vi "callTransport.vi"() -> ()   [LabVIEW 2019]
uses:
  <userlib>/LevyLab/Transport/Control Experiment/Control Experiment.lvclass/Control Experiment.ctl
  <userlib>/LevyLab/Transport/Transport/Transport.lvclass/Transport.ctl
  <userlib>/LevyLab/Transport/Transport/Transport.lvclass
  <userlib>/LevyLab/Transport/Control Experiment/Control Experiment.lvclass
  <vilib>/Wiresmith Technology/G CLI/CLI Class/CLI.lvclass
panel:
  out "TDMS Params":cluster{"Key":string, "Value":dbl}[](array[cluster])
  out "Comments":string
  out "Experiment Folder":string
  out "Calling VI":string
  # "[FLEX <-> callTransport]"
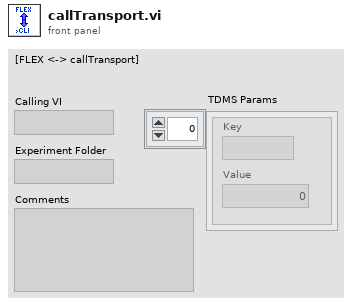
[diagram p1: front panel]
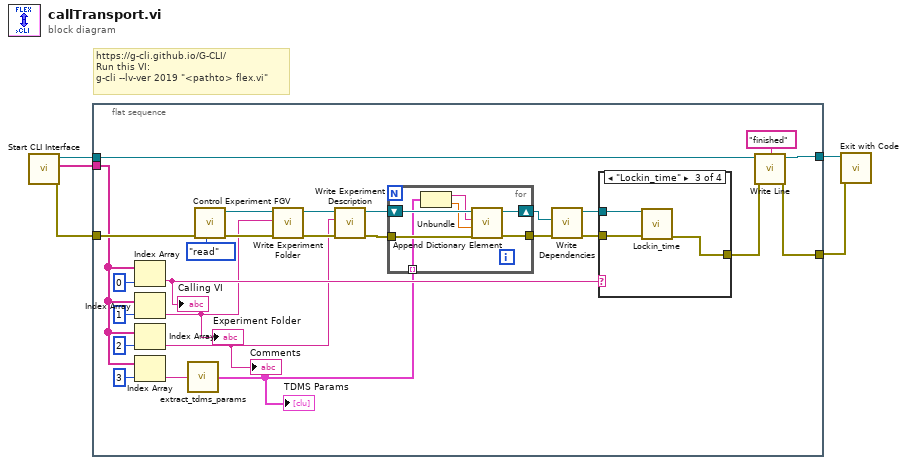
[diagram p0: block diagram]
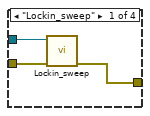
[diagram p2: hidden frame]
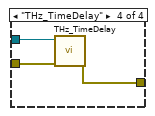
[diagram p4: hidden frame]
diagram:
  # "https://g-cli.github.io/G-CLI/\nRun this VI:\ng-cli --lv-ver 2019 \"<pathto> flex.vi\""
  n1 = call <vilib>:"Start CLI Interface.vi"() -> ("error out"=w5:errorcluster, "Custom Parameters"=w1:string[], "CLI out"=w4:refnum<class "CLI.lvclass">)  [unwired: 8 in, 1 out]
  n2 = flat-sequence {
    tunnel: w5 -> [w29]
    tunnel: w4 -> [w27]
    tunnel: [w26] -> w3
    tunnel: [w25] -> w2
    tunnel: w1 -> [w10]
    frame #0 {
      n3 = Index Array(array=w10, index=0) -> (element=w9:string)
      "Calling VI" <- w9
      n4 = Index Array(array=w10, index=1) -> (element=w8:string)
      "Experiment Folder" <- w8
      n5 = Index Array(array=w10, index=2) -> (element=w7:string)
      "Comments" <- w7
      n6 = Index Array(array=w10, index=3) -> (element=w13:string)
      n7 = call "extract_tdms_params.vi"("Input String"=w13) -> ("Output Array"=w6:cluster{"key":string, "value":dbl}[])
      "TDMS Params" <- w6
      n8 = call <userlib>:"Control Experiment FGV.vi"("Function"=enum16{"read", "write"}."read", "error in (no error)"=w29) -> ("error out"=w21:errorcluster, "Control Experiment.lvclass out"=w23:refnum<class "Control Experiment.lvclass">)  [unwired: 8 in]
      n9 = call <userlib>:"Write Experiment Folder.vi"("error in (no error)"=w21, "Experiment Folder"=w8, "Control Experiment in"=w23) -> ("error out"=w20:errorcluster, "Control Experiment out"=w22:refnum<class "Control Experiment.lvclass">)  [unwired: 7 in]
      n10 = call <userlib>:"Write Experiment Description.vi"("error in (no error)"=w20, "Experiment Description"=w7, "Control Experiment in"=w22) -> ("error out"=w14:errorcluster, "Control Experiment out"=w17:refnum<class "Control Experiment.lvclass">)  [unwired: 7 in]
      n11 = for {
        shift-right: [w49] -> w16
        shift-left: w17 -> [w48]
        tunnel: [w47] -> w15
        tunnel: w14 -> [w46]
        tunnel: w6 -> [w45] mode=indexing
        n12 = Unbundle(w45) -> ("key"=w44:string, "value"=w43:dbl)
        n13 = call <userlib>:"Append Dictionary Element.vi"("error in (no error)"=w46, "value"=w43, "key"=w44, "Control Experiment in"=w48) -> ("error out"=w47:errorcluster, "Control Experiment out"=w49:refnum<class "Control Experiment.lvclass">)  [unwired: 6 in]
      }
      n14 = call <userlib>:"Write Dependencies.vi"("error in (no error)"=w15, "Control Experiment"=w16) -> ("error out"=w30:errorcluster, "Transport out"=w31:refnum<class "Transport.lvclass">)  [unwired: 8 in]
      n15 = case shown="\"Lockin_time\"" w9 {
        tunnel: w31 -> [w35 _ w39 w42]
        tunnel: w30 -> [w34 w36 w38 w41]
        tunnel: [w33 w36 w37 w40] -> w24
        frame "Lockin_sweep" {
          n16 = call <userlib>:"Lockin_sweep.vi"("Transport"=w35, "error in (no error)"=w34) -> ("error out"=w33:errorcluster)  [unwired: 7 in, 1 out]
        }
        frame Default {
        }
        frame "Lockin_time" {
          n17 = call <userlib>:"Lockin_time.vi"("error in (no error)"=w38, "Transport"=w39) -> ("error out"=w37:errorcluster)  [unwired: 8 in, 1 out]
        }
        frame "THz_TimeDelay" {
          n18 = call <userlib>:"THz_TimeDelay.vi"("error in (no error)"=w41, "Transport"=w42) -> ("error out"=w40:errorcluster)  [unwired: 8 in, 1 out]
        }
      }
      n19 = call <vilib>:"Write Line.vi"("error in (no error)"=w24, "Text to Write"="finished", "CLI in"=w27) -> ("error out"=w25:errorcluster, "CLI out"=w26:refnum<class "CLI.lvclass">)  [unwired: 7 in]
    }
  }
  n20 = call <vilib>:"Exit with Code.vi"("error in (no error)"=w2, "CLI in"=w3) -> ()  [unwired: 9 in, 1 out]
